vi "Find Closest Point In Path.vi"(1 "Length":dbl, 2 "Points":T2(array[cluster])) -> (0 "Point":T1={"X"=43.916679291641024, "Y"=47.99228927660444, "Theta[rad]"=3.068267674373451, "R"=-18.560947731190943, "Length"=47.539190662540875, "s"=0.8282828282828283})   [LabVIEW 2015]
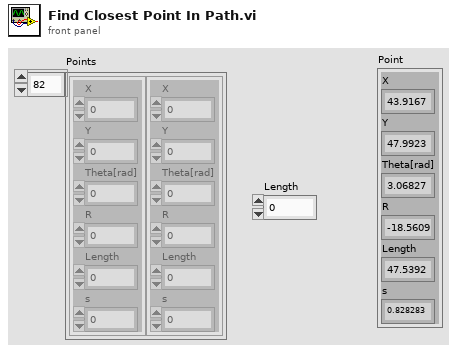
[diagram p1: front panel]
types:
  T1 = cluster{"X":dbl, "Y":dbl, "Theta[rad]":dbl, "R":dbl, "Length":dbl, "s":dbl}
  T2 = cluster{"X":dbl, "Y":dbl, "Theta[rad]":dbl, "R":dbl, "Length":dbl, "s":dbl}[]
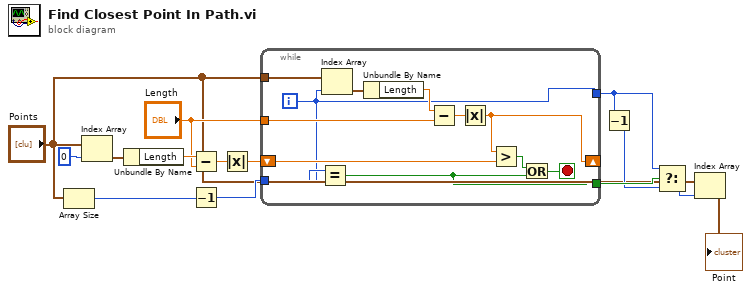
[diagram p0: block diagram]
diagram:
  n1 = Array Size(array="Points") -> (size(s)=w14:i32)
  n2 = Index Array(array="Points", index=0) -> (element=w11:T1)
  n3 = Unbundle By Name(w11) -> ("Length"=w9:dbl)
  n4 = Subtract(x=w9, y="Length") -> (x-y=w10:dbl)
  n5 = Decrement(x=w14) -> (x-1=w13:i32)
  n6 = Absolute Value(x=w10) -> (abs(x)=w7:dbl)
  n7 = while {
    tunnel: w13 -> [w26]
    tunnel: "Points" -> [w25]
    tunnel: "Length" -> [w22]
    shift-right: [w17] -> _
    shift-left: w7 -> [w20]
    tunnel: [w16] -> w5
    tunnel: [w15] -> w6
    i -> [w16]
    stop <- w19 stop-if-true
    n8 = Equal?(x=w26, y=w16) -> (x = y?=w15:bool)
    n9 = Index Array(array=w25, index=w16) -> (element=w24:T1)
    n10 = Unbundle By Name(w24) -> ("Length"=w23:dbl)
    n11 = Subtract(x=w23, y=w22) -> (x-y=w21:dbl)
    n12 = Absolute Value(x=w21) -> (abs(x)=w17:dbl)
    n13 = Greater?(x=w17, y=w20) -> (0:w18:bool)
    n14 = Or(x=w18, y=w15) -> (x .or. y?=w19:bool)
  }
  n15 = Decrement(x=w5) -> (x-1=w4:i32)
  n16 = Select(t=w5, s=w6, f=w4) -> (s? t:f=w2:i32)
  n17 = Index Array(array="Points", index=w2) -> (element=→"Point":T1)
